vi "Write data to DB.vi"(8 "error in (no error)":errorcluster, 9 "Procedure name":string, 10 "all string":string, 11 "DSN name":string) -> (0 "error out":errorcluster, 2 "ResultA":string, 3 "FSNA":string)   [LabVIEW 2013]
uses:
  <vilib>/addons/database/Connection.llb/DB Tools Open Connec (String).vi
  <vilib>/addons/database/Connection.llb/Conn Execute.vi
  <vilib>/addons/database/Recordset.llb/Rec Fetch Recordset Data (R).vi
  <vilib>/addons/database/Recordset.llb/Rec Destroy - Connection.vi
  <vilib>/addons/database/NI_Database_API.lvlib
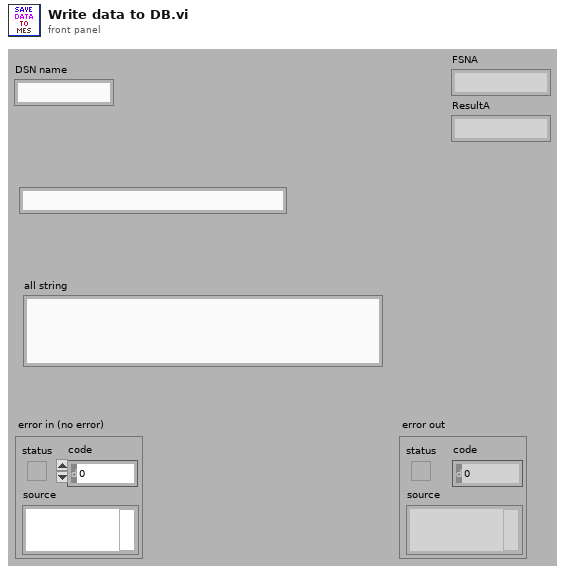
[diagram p1: front panel]
types:
  T1 = typedef "NI_Database_API.lvlib/Conn ObjectReference.ctl" = refnum<k1>
  T2 = typedef "NI_Database_API.lvlib/Rec ObjectReference.ctl" = refnum<k1>
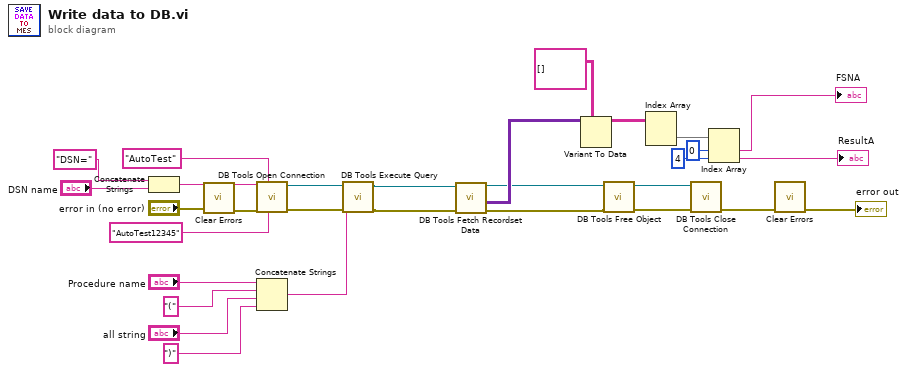
[diagram p0: block diagram]
diagram:
  n1 = Concatenate Strings("DSN=", "DSN name") -> (w20:string)
  n2 = call <vilib>:"Clear Errors.vi"("error in (no error)"="error in (no error)") -> ("error out"=w1:errorcluster)  [unwired: 6 in]
  n3 = call-poly <vilib>:"DB Tools Open Connection.vi"("password"="AutoTest12345" ("userID"), "userID"="AutoTest", "error in (no error)"=w1, "connection information"=w20) -> ("error out"=w30:errorcluster, "connection reference"=w29:T1)  [unwired: 4 in]
  n4 = Concatenate Strings("Procedure name", "(", "all string", ")") -> (w25:string)
  n5 = call-poly <vilib>:"DB Tools Execute Query.vi"("error in (no error)"=w30, "SQL query"=w25, "connection reference"=w29) -> ("error out"=w13:errorcluster, "recordset reference"=w14:T2)  [unwired: 5 in]
  n6 = call-poly <vilib>:"DB Tools Fetch Recordset Data.vi"("error in (no error)"=w13, "recordset reference"=w14) -> ("error out"=w11:errorcluster, "recordset data"=w16:variant[][], "recordset reference out"=w12:T2)  [unwired: 3 in]
  n7 = Variant To Data(type=string[][] [], Variant=w16) -> (data=w10:string[][])  [unwired: 1 in, 1 out]
  n8 = call-poly <vilib>:"DB Tools Free Object.vi"("error in (no error)"=w11, "recordset reference"=w12) -> ("error out"=w27:errorcluster, "connection reference"=w28:T1)  [unwired: 8 in]
  n9 = Index Array(array=w10) -> (element=w9:string[])  [unwired: 2 in]
  n10 = call <vilib>:"DB Tools Close Connection.vi"("error in (no error)"=w27, "connection reference"=w28) -> ("error out"=w4:errorcluster)  [unwired: 5 in]
  n11 = Index Array(array=w9, index #1=0 ("索引"), index #2=4 ("索引")) -> (element #1=→"FSNA":string, element #2=→"ResultA":string)
  n12 = call <vilib>:"Clear Errors.vi"("error in (no error)"=w4) -> ("error out"=→"error out":errorcluster)  [unwired: 6 in]
